vi "yolov9_openvino_camera.vi"() -> ()   [LabVIEW 2018]
uses:
  <vilib>/addons/VIRobotics/ModelZoo/Object_Detection/yolov8_openvino/InitialModel_yolov9_OpenVINO_IR.vi
  <vilib>/addons/VIRobotics/opencv_yiku/Cap/Cap.lvclass
  <vilib>/addons/VIRobotics/ModelZoo/Object_Detection/yolov8_openvino/yolov8_openvino.lvclass
panel:
  in  "Frame_Height":dbl=720.0 format="%#_13g"
  in  "Frame_Width":dbl=1280.0 format="%#_13g"
  in  "cameraID":i32
  in  "device_name":string(combo)="CPU"
  out "每帧耗时(s)":dbl
  in  "stop":bool
  out "picture":picture
  # "yolov9c OpenVINO 1280*720 on LabVIEW"
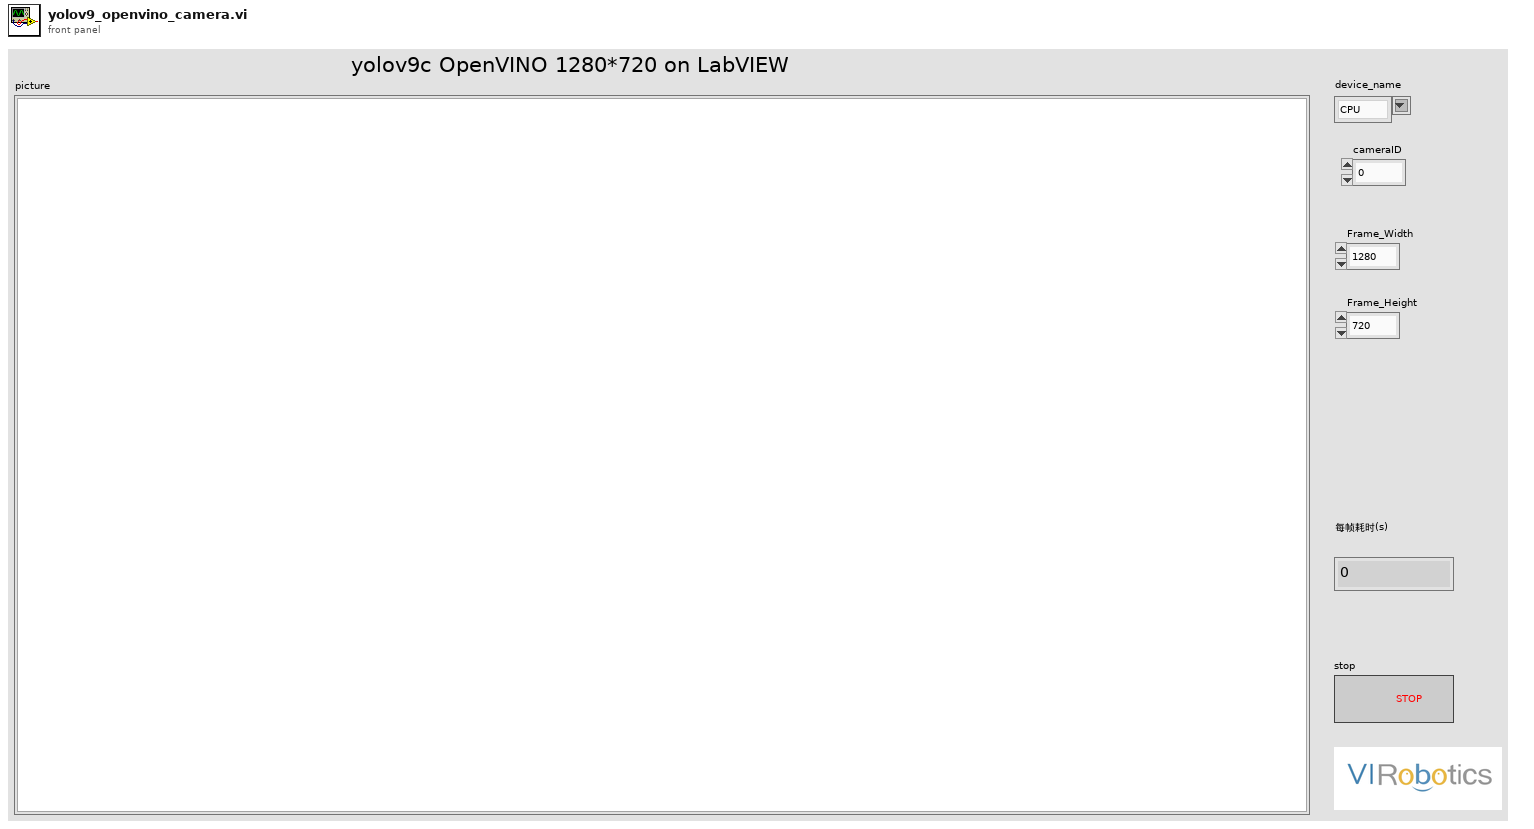
[diagram p1: front panel]
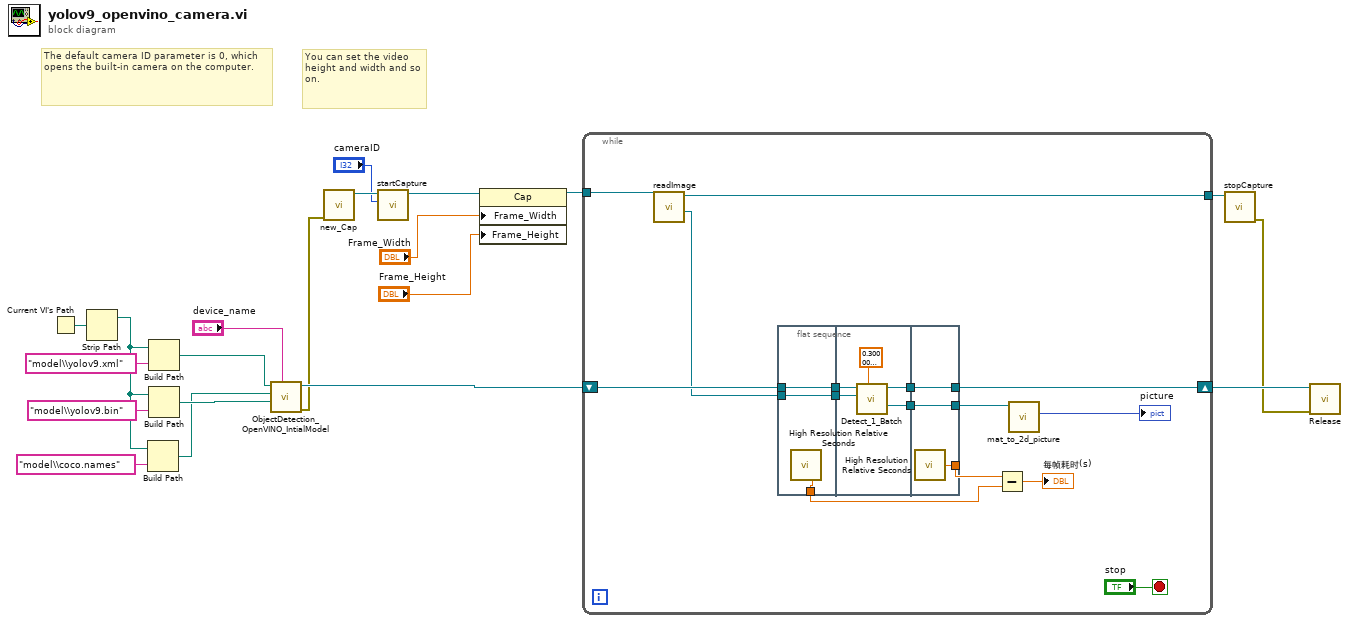
[diagram p0: block diagram]
diagram:
  # "You can set the video height and width and so on."
  # "The default camera ID parameter is 0, which opens the built-in camera on the computer."
  n1 = Current VI's Path() -> (path=w15:path)
  n2 = Strip Path(path=w15) -> (stripped path=w8:path)  [unwired: 1 out]
  n3 = Build Path(base path=w8, name or relative path="model\\coco.names") -> (appended path=w9:path)
  n4 = Build Path(base path=w8, name or relative path="model\\yolov9.xml") -> (appended path=w12:path)
  n5 = Build Path(base path=w8, name or relative path="model\\yolov9.bin") -> (appended path=w11:path)
  n6 = call-poly <vilib>:"ObjectDetection_OpenVINO_IntialModel.vi"("device_name"="device_name", "bin_fle"=w11, "class_names_path"=w9, "xmlPath"=w12) -> ("error out"=w2:errorcluster, "yolov9_openvino out"=w17:refnum<class "yolov8_openvino.lvclass">)  [unwired: 6 in]
  n7 = call <vilib>:"new_Cap.vi"("error in (no error)"=w2) -> ("Cap out"=w7:refnum<class "Cap.lvclass">)  [unwired: 9 in, 1 out]
  n8 = call <vilib>:"startCapture.vi"("cameraID"="cameraID", "Cap in"=w7) -> ("Cap out"=w4:refnum<class "Cap.lvclass">)  [unwired: 8 in, 1 out]
  n9 = property class="Cap"(reference=w4, "Frame_Width"="Frame_Width", "Frame_Height"="Frame_Height") -> (reference out=w1:refnum<class "Cap.lvclass">)  [unwired: 1 in, 1 out]
  n10 = while {
    shift-right: [w32] -> w19
    shift-left: w17 -> [w35]
    tunnel: [w31] -> w20
    tunnel: w1 -> [w21]
    stop <- "stop" stop-if-true
    n11 = call <vilib>:"readImage.vi"("Cap in"=w21) -> ("Mat out"=w24:refnum<class "Mat_8U.lvclass">, "Cap out"=w31:refnum<class "Cap.lvclass">)  [unwired: 8 in, 1 out]
    n12 = flat-sequence {
      tunnel: w35 -> [w38]
      tunnel: [w38] -> w30
      tunnel: [w37] -> w26
      tunnel: w24 -> [w36]
      tunnel: [w36] -> w23
      tunnel: w30 -> [w43]
      tunnel: [w42] -> w29
      tunnel: [w41] -> w28
      tunnel: w23 -> [w40]
      tunnel: [w45] -> w32
      tunnel: [w46] -> w34
      tunnel: w29 -> [w46]
      tunnel: w28 -> [w45]
      tunnel: [w44] -> w27
      frame #0 {
        n13 = call <vilib>:"High Resolution Relative Seconds.vi"() -> ("relative seconds"=w37:dbl)
      }
      frame #1 {
        n14 = call-dynamic "Detect_1_Batch.vi"("confThreshold"=sgl 0.3, "image"=w40, "yolov8_openvino in"=w43) -> ("img out"=w42:refnum<class "Mat_8U.lvclass">, "yolov8_openvino out"=w41:refnum<class "yolov8_openvino.lvclass">)  [unwired: 5 in, 2 out]
      }
      frame #2 {
        n15 = call <vilib>:"High Resolution Relative Seconds.vi"() -> ("relative seconds"=w44:dbl)
      }
    }
    n16 = Subtract(x=w27, y=w26) -> (x-y=→"每帧耗时(s)":dbl)
    n17 = call <vilib>:"mat_to_2d_picture.vi"("Mat_8U in"=w34) -> ("picture"=→"picture":picture)  [unwired: 8 in, 2 out]
  }
  n18 = call <vilib>:"stopCapture.vi"("Cap in"=w20) -> ("error out"=w18:errorcluster)  [unwired: 10 in]
  n19 = call-dynamic "Release.vi"("error in (no error)"=w18, "yolov8_openvino in"=w19) -> ()  [unwired: 8 in, 2 out]
